vi "Component Loader Error Info.vi"(11 "error":T1) -> (3 "error info":cluster{"code":i32, "description":string})   [LabVIEW 2020, in "DSF Core.lvlib" / "Component Loader.lvclass"]
uses:
  Component Loader.lvclass
  Framework/Framework.lvclass
  VIs/Constants/Base Error Code.vi
  Errors.ctl
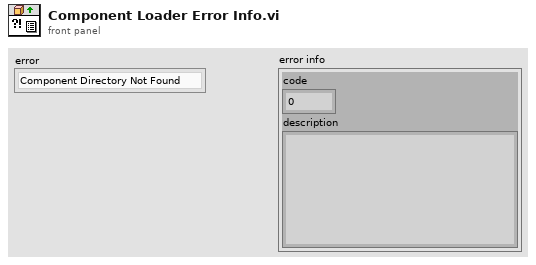
[diagram p1: front panel]
types:
  T1 = typedef "DSF Core.lvlib/Component Loader.lvclass/Errors.ctl" = enum16{"Component Directory Not Found", "Component Not Found", "Class Not Found"}
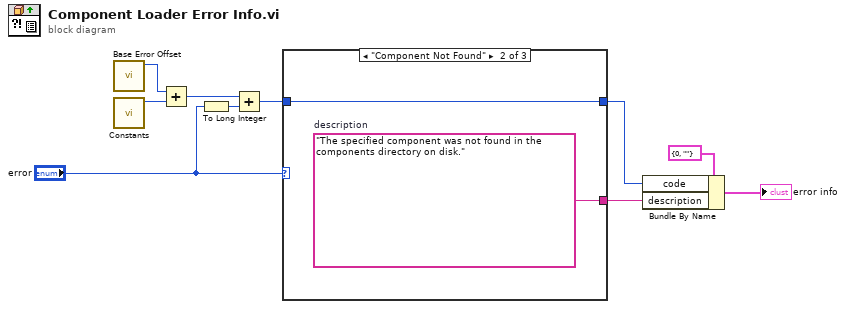
[diagram p0: block diagram]
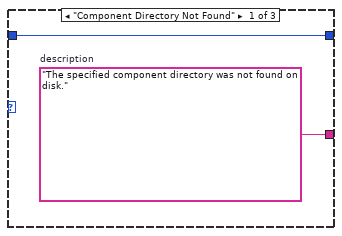
[diagram p2: hidden frame]
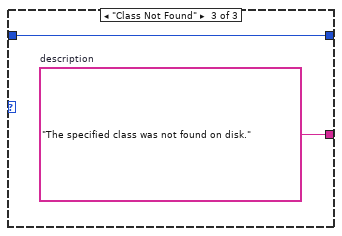
[diagram p3: hidden frame]
diagram:
  n1 = call "Base Error Offset.vi"() -> ("base error offset"=w10:i32)  [unwired: 11 in]
  n2 = call-poly "Constants.vi"() -> ("base error code"=w9:i32)  [unwired: 11 in]
  n3 = Add(x=w10, y=w9) -> (x+y=w3:i32)
  n4 = To Long Integer(number="error") -> (32bit integer=w8:i32)
  n5 = Add(x=w3, y=w8) -> (x+y=w2:i32)
  n6 = case shown="\"Component Not Found\"" "error" {
    tunnel: [w12 w14 w16] -> w5
    tunnel: w2 -> [w11 w13 w15]
    tunnel: [w11 w13 w15] -> w1
    frame "Component Directory Not Found" {
      w12 = "The specified component directory was not found on disk."  # description
    }
    frame "Component Not Found" {
      w14 = "The specified component was not found in the components directory on disk."  # description
    }
    frame "Class Not Found" {
      w16 = "The specified class was not found on disk."  # description
    }
  }
  n7 = Bundle By Name(cluster=cluster{"code":i32, "description":string} {"code"=0, "description"=""}, "code"=w1, "description"=w5) -> (→"error info":cluster{"code":i32, "description":string})
